vi "Write Y.vi"(8 "error in (no error)":errorcluster, 10 "Y":cdb[](array[numeric]), 11 "Y (1Ch) in":refnum<class "Y (Complex) (1 Ch).lvclass">) -> (0 "error out":errorcluster, 3 "Y (1Ch) out":refnum<class "Y (Complex) (1 Ch).lvclass">)   [LabVIEW 2017, in "Y (Complex) (1 Ch).lvclass"]
uses:
  <vilib>/addons/_NISVFA/_Shared subVIs/Data Objects/Y (Complex) (DBL)/Y (Complex) (1 Ch).lvclass
  <vilib>/addons/_NISVFA/_Shared subVIs/Data Objects/Y (Complex) (DBL)/Y (Complex) (1 Ch).lvclass/Y (Complex) (1 Ch).ctl
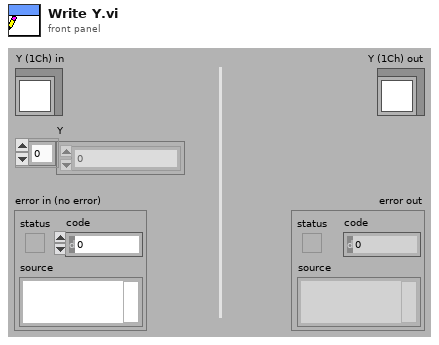
[diagram p1: front panel]
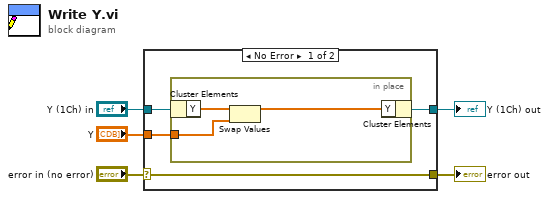
[diagram p0: block diagram]
diagram:
  n1 = case shown="No Error" "error in (no error)" {
    selector: "error in (no error)" -> [w9 w13]
    tunnel: [w9 w13] -> w4
    tunnel: [w7 w14] -> w2
    tunnel: "Y (1Ch) in" -> [w8 w14]
    tunnel: "Y" -> [w6 _]
    frame No Error {
      n2 = in-place {
        in-place-border: w6 -> [w11]
        n3 = in-place-cluster #1(w8) -> ("Y"=w12:cdb[])
        n4 = Swap Values(12:w12, 14:w11) -> (1:w10:cdb[])  [unwired: 1 in, 1 out]
        n5 = in-place-cluster #1("Y"=w10) -> (w7:refnum<class "Y (Complex) (1 Ch).lvclass">)
      }
    }
    frame Error {
    }
  }
  "error out" <- w4
  "Y (1Ch) out" <- w2
